vi "Calling VI.vi"   [LabVIEW 2023]
doc: "This VI is not a member of any LabVIEW class and has no special access privileges such as friendship with a class."
uses:
  Class A/Class A.lvclass
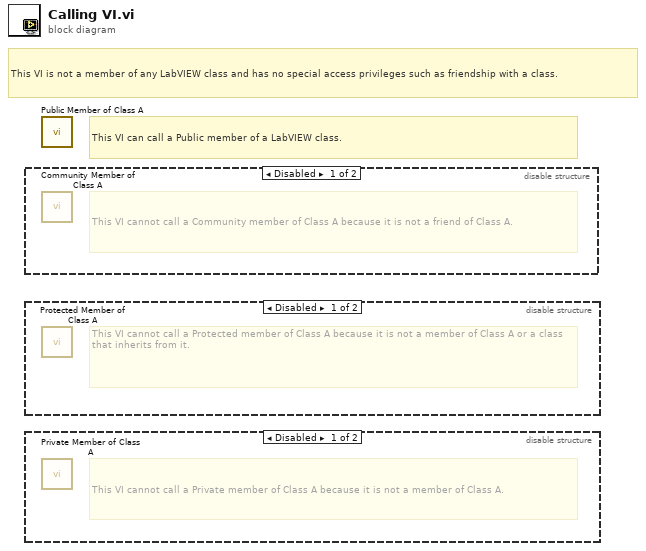
[diagram p0: block diagram]
diagram:
  # "This VI can call a Public member of a LabVIEW class."
  # "This VI is not a member of any LabVIEW class and has no special access privileges such as friendship with a class."
  n1 = disable-structure shown="Disabled" {
    frame Disabled {
      # "This VI cannot call a Community member of Class A because it is not a friend of Class A."
      n2 = call "Community Member of Class A.vi"() -> ()  [unwired: 12 in]
    }
    frame Enabled {
    }
  }
  n3 = disable-structure shown="Disabled" {
    frame Disabled {
      # "This VI cannot call a Protected member of Class A because it is not a member of Class A or a class that inherits from it."
      n4 = call "Protected Member of Class A.vi"() -> ()  [unwired: 12 in]
    }
    frame Enabled {
    }
  }
  n5 = disable-structure shown="Disabled" {
    frame Disabled {
      # "This VI cannot call a Private member of Class A because it is not a member of Class A."
      n6 = call "Private Member of Class A.vi"() -> ()  [unwired: 12 in]
    }
    frame Enabled {
    }
  }
  n7 = call "Public Member of Class A.vi"() -> ()  [unwired: 12 in]
